vi "mav_msg_read.vi"(8 "error in":errorcluster, 9 "Connection Type":enum32{"TCP", "SERIAL", "UDP"}(tab), 11 "mav_connection_in":T1) -> (0 "error out":errorcluster, 2 "mav_msg":T3, 3 "mav_connection_out":T1)   [LabVIEW 2023]
panel:
  out "crc_counter":u32
  out "packet_counter":u32
  out "mav_msg_array":T2(array[cluster])
  out "check_mav_msg_array":bool
  out "CRC":bool
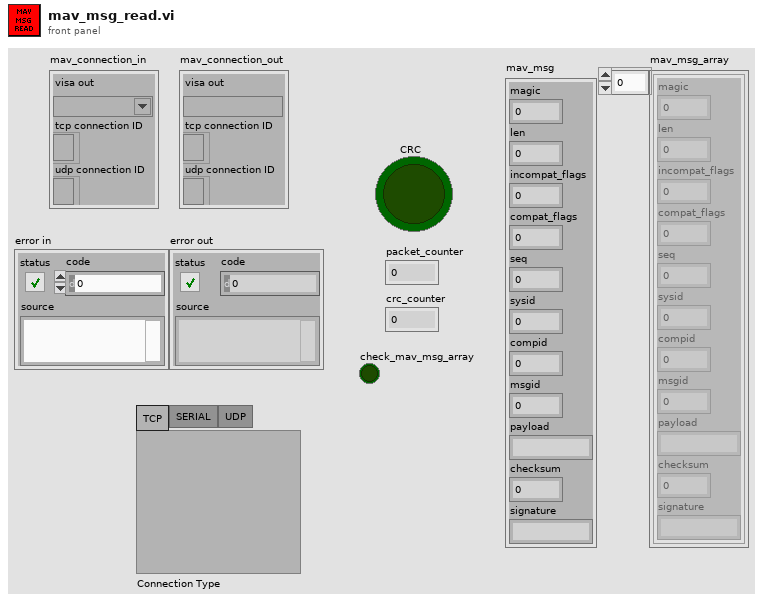
[diagram p1: front panel]
types:
  T1 = cluster{"visa out":refnum<visa-resource-name>, "tcp connection ID":refnum<k5>, "udp connection ID":refnum<k16>}
  T2 = cluster{"len":u8, "incompat_flags":u8, "compat_flags":u8, "seq":u8, "sysid":u8, "compid":u8, "msgid":u32, "magic":u8, "payload":string, "checksum":u16, "signature":string}[]
  T3 = cluster{"len":u8, "incompat_flags":u8, "compat_flags":u8, "seq":u8, "sysid":u8, "compid":u8, "msgid":u32, "magic":u8, "payload":string, "checksum":u16, "signature":string}
  T4 = cluster{"VISA out":refnum<visa-resource-name>, "tcp connection ID":refnum<k5>, "udp connection ID":refnum<k16>}
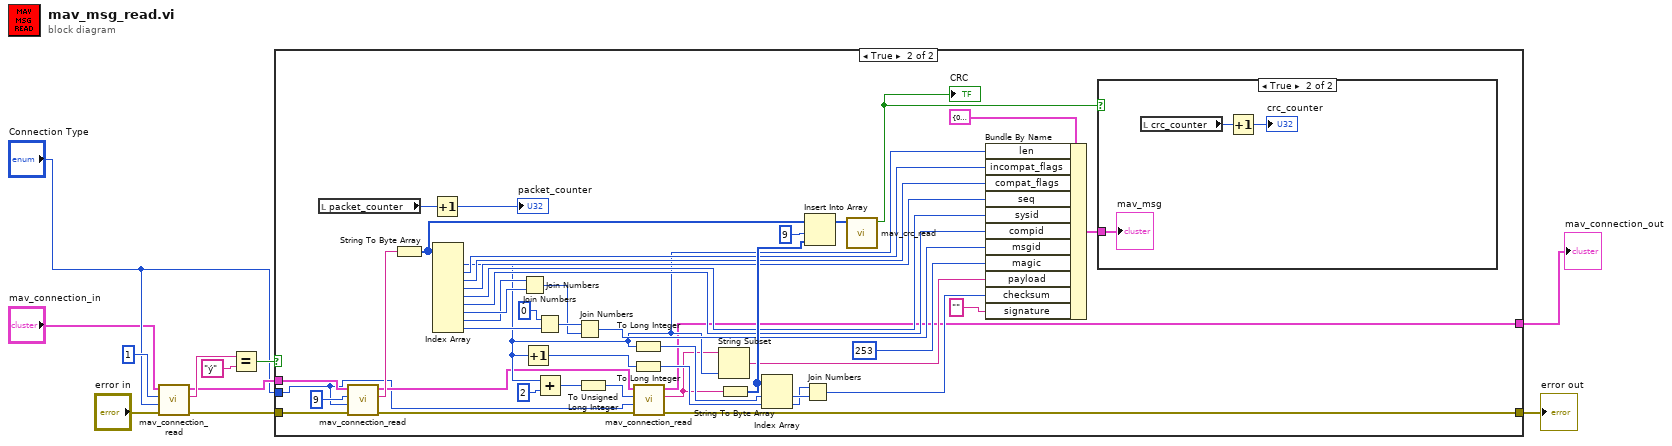
[diagram p0: block diagram]
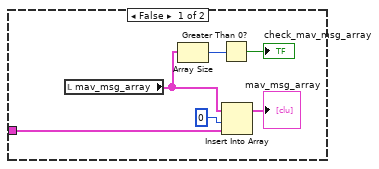
[diagram p3: hidden frame]
diagram:
  n1 = call "mav_connection_read.vi"("error in"="error in", "Connection Type"="Connection Type", "bytes to read"=u32 1 ("byte count"), "mav_connection_in"="mav_connection_in") -> ("error out"=w6:errorcluster, "data out"=w7:string, "mav_connection_out"=w5:T4)  [unwired: 5 in]
  n2 = Equal?(x=w7, y="ý") -> (x = y?=w11:bool)
  n3 = case shown="True" w11 {
    tunnel: w5 -> [w12 w24]
    tunnel: w6 -> [w13 w23]
    tunnel: [w13 w16] -> w4
    tunnel: [w12 w17] -> w2
    tunnel: "Connection Type" -> [_ w14]
    frame False {
    }
    frame True {
      n4 = local read "packet_counter"() -> (w57:u32)
      n5 = call "mav_connection_read.vi"("error in"=w23, "Connection Type"=w14, "bytes to read"=u32 9 ("byte count"), "mav_connection_in"=w24) -> ("error out"=w18:errorcluster, "data out"=w20:string, "mav_connection_out"=w19:T4)  [unwired: 5 in]
      n6 = String To Byte Array(string=w20) -> (unsigned byte array=w43:u8[])
      n7 = Increment(x=w57) -> (x+1=→"packet_counter":u32)
      n8 = Index Array(array=w43) -> (element #1=w25:u8, element #2=w37:u8, element #3=w36:u8, element #4=w35:u8, element #5=w34:u8, element #6=w33:u8, element #7=w53:u8, element #8=w52:u8, element #9=w51:u8)  [unwired: 9 in]
      n9 = Join Numbers(hi=w52, lo=w53) -> ((hi.lo)=w48:u16)
      n10 = Increment(x=w25) -> (x+1=w45:u8)
      n11 = Join Numbers(hi=u8 0, lo=w51) -> ((hi.lo)=w49:u16)
      n12 = Add(x=w25, y=u8 2) -> (x+y=w47:u8)
      n13 = Join Numbers(hi=w49, lo=w48) -> ((hi.lo)=w32:u32)
      n14 = To Unsigned Long Integer(number=w47) -> (unsigned 32bit integer=w21:u32)
      n15 = To Long Integer(number=w25) -> (32bit integer=w44:i32)
      n16 = To Long Integer(number=w45) -> (32bit integer=w46:i32)
      n17 = call "mav_connection_read.vi"("error in"=w18, "Connection Type"=w14, "bytes to read"=w21, "mav_connection_in"=w19) -> ("error out"=w16:errorcluster, "data out"=w15:string, "mav_connection_out"=w17:T4)  [unwired: 5 in]
      n18 = String Subset(string=w15, length (rest)=w25) -> (substring=w31:string)  [unwired: 1 in]
      n19 = String To Byte Array(string=w15) -> (unsigned byte array=w42:u8[])
      n20 = Index Array(array=w42, index #1=w44, index #2=w46) -> (element #1=w41:u8, element #2=w40:u8)
      n21 = Join Numbers(hi=w40, lo=w41) -> ((hi.lo)=w30:u16)
      n22 = Insert Into Array(array=w43, index=9, new element=w42) -> (w56:u8[])
      n23 = call "mav_crc_read.vi"("byte_array_in"=w56) -> ("CRC"=w39:bool)  [unwired: 10 in]
      "CRC" <- w39
      n24 = Bundle By Name(cluster=T3 {"len"=0, "incompat_flags"=0, "compat_flags"=0, "seq"=0, "sysid"=0, "compid"=0, "msgid"=0, "magic"=0, "payload"="", "checksum"=0, "signature"=""} ("mav_msg"), "len"=w25, "incompat_flags"=w37, "compat_flags"=w36, "seq"=w35, "sysid"=w34, "compid"=w33, "msgid"=w32, "magic"=u8 253, "payload"=w31, "checksum"=w30, "signature"="") -> (w26:T3)
      n25 = case shown="True" w39 {
        tunnel: w26 -> [w62 w66]
        frame False {
          n26 = local read "mav_msg_array"() -> (w60:T2)
          n27 = Array Size(array=w60) -> (size(s)=w61:i32)
          n28 = Greater Than 0?(x=w61) -> (x > 0?=→"check_mav_msg_array":bool)
          n29 = Insert Into Array(array=w60, index=0, new element=w62) -> (→"mav_msg_array":T2)
        }
        frame True {
          n30 = local read "crc_counter"() -> (w65:u32)
          n31 = Increment(x=w65) -> (x+1=→"crc_counter":u32)
          "mav_msg" <- w66
        }
      }
    }
  }
  "error out" <- w4
  "mav_connection_out" <- w2
